vi "GetInterface.vi"(3 "error in":errorcluster) -> (0 "VISA resource name":refnum<visa-resource-name>, 6 "error out":errorcluster)   [LabVIEW 2011]
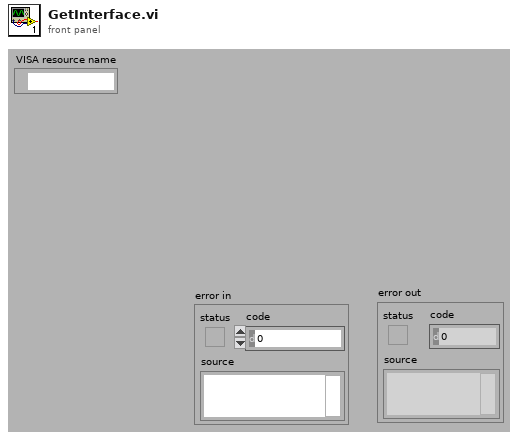
[diagram p1: front panel]
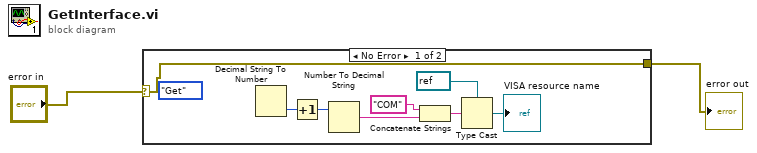
[diagram p0: block diagram]
diagram:
  n1 = case shown="No Error" "error in" {
    selector: "error in" -> [w3 w12]
    tunnel: [w3 w12] -> w1
    frame No Error {
      w10 = enum16{"Set", "Get"}."Get" ("Set_Get")
      n2 = Decimal String To Number() -> (number=w7:i32)  [unwired: 3 in, 1 out]
      n3 = Increment(x=w7) -> (x+1=w8:i32)
      n4 = Number To Decimal String(number=w8) -> (decimal integer string=w9:string)  [unwired: 1 in]
      n5 = Concatenate Strings("COM" ("string"), w9) -> (w6:string)
      n6 = Type Cast(type=refnum<visa-resource-name> refnum ("VISA resource name"), x=w6) -> (*(type *) &x=→"VISA resource name":refnum<visa-resource-name>)
    }
    frame Error {
    }
  }
  "error out" <- w1
